vi "GUI AC Source setup.vi"(11 "AC Source":T2) -> (3 "AC Source out":T2)   [LabVIEW 2020]
doc: "Use this template to build a producer/consumer design pattern with events to produce queue items. Use this design pattern instead of the User Interface Event Handler pattern for user interfaces when you want to execute code asynchronously in response to an event without slowing the user interface responsiveness."
uses:
  General AC source/Type definitions/AC Source.ctl
  General AC source/Type definitions/AC Source type.ctl
  <vilib>/Utility/error.llb/DialogType.ctl
  <vilib>/Utility/error.llb/Error Cluster From Error Code.vi
  <vilib>/ErrorRing/Error Ring.xnode
  external libraries/varilib/varilib.lvlib
panel:
  out "not tested label":string="This device is not\nyet fully tested!"
  in  "Ref. clock (Hz)":dbl caption="Reference clock (Hz)\nIf set to zero, ref. clock is not used." format="%#_6p"
  in  "AC source type":T1
  in  "VISA":refnum<visa-resource-name>
  out "gui_elements":refnum<vi>[](array[refnum])
  out "Status":string
  in  "save_and_quit":bool
  in  "test":bool
  in  "cancel":bool
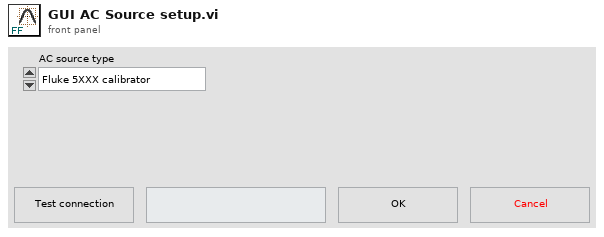
[diagram p1: front panel]
types:
  T1 = typedef "AC Source type.ctl" = enum16{"Fluke 5XXX calibrator", "Tektronix AFG3101C", "dummy"}
  T2 = typedef "AC Source.ctl" = cluster{"AC Source type":T1, "VISA":refnum<visa-resource-name>, "Ref. clock (Hz)":dbl, "status ref":refnum<vi>}
  T3 = typedef "DialogType.ctl" = u16
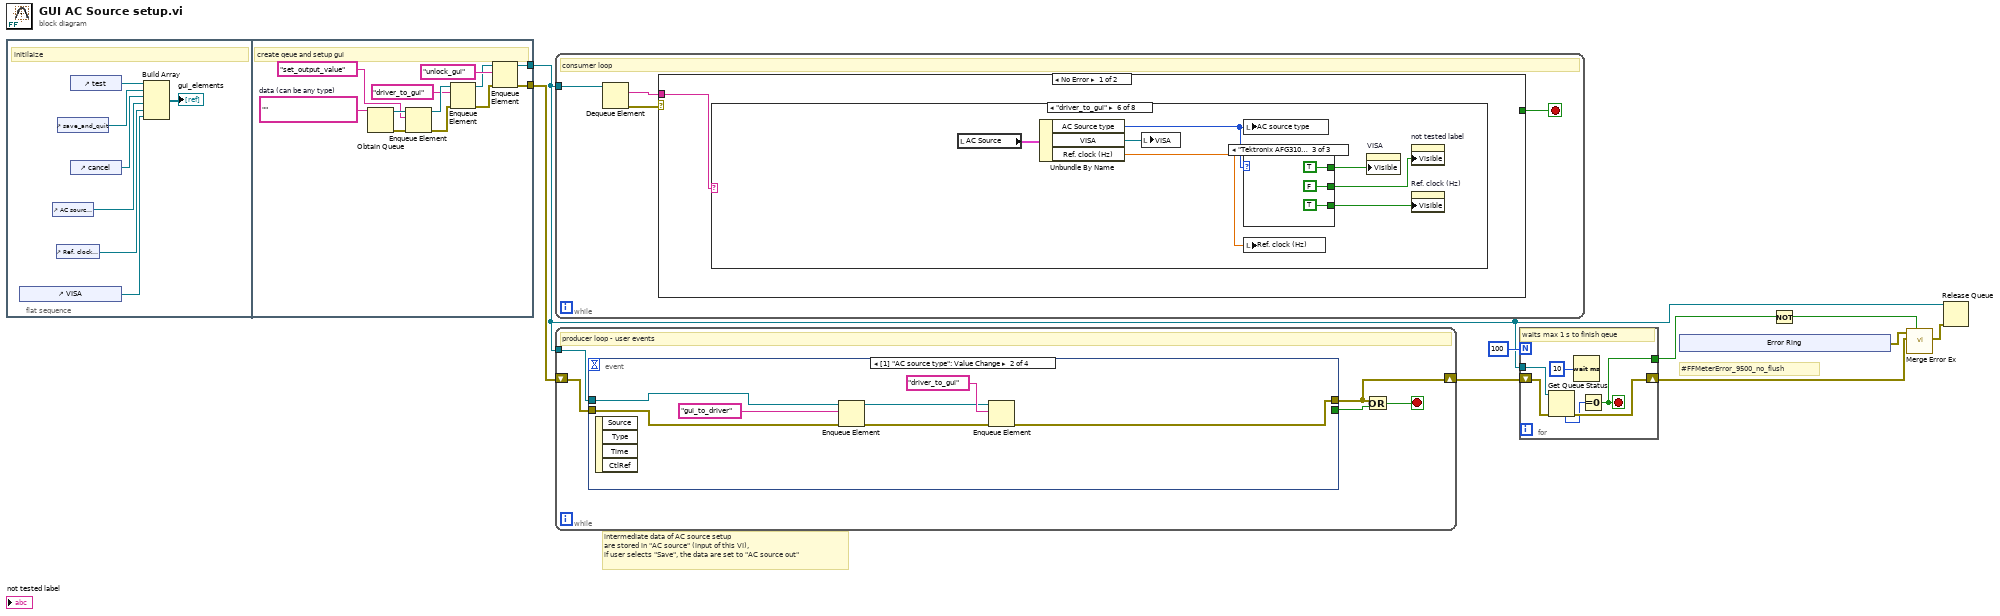
[diagram p0: block diagram]
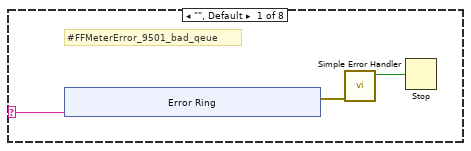
[diagram p2: hidden frame]
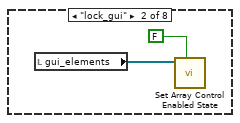
[diagram p3: hidden frame]
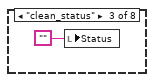
[diagram p4: hidden frame]
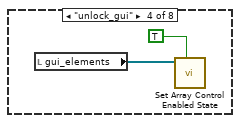
[diagram p5: hidden frame]
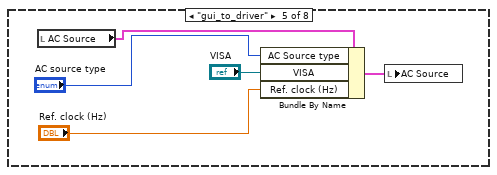
[diagram p6: hidden frame]
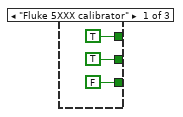
[diagram p7: hidden frame]
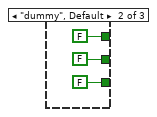
[diagram p8: hidden frame]
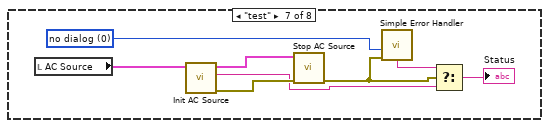
[diagram p9: hidden frame]
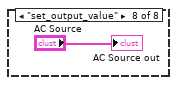
[diagram p10: hidden frame]
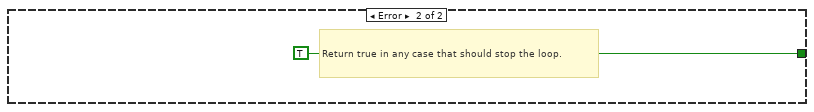
[diagram p11: hidden frame]
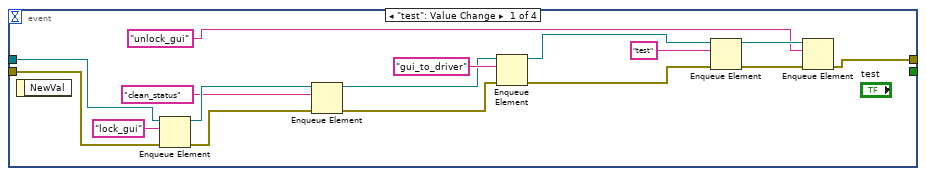
[diagram p12: hidden frame]
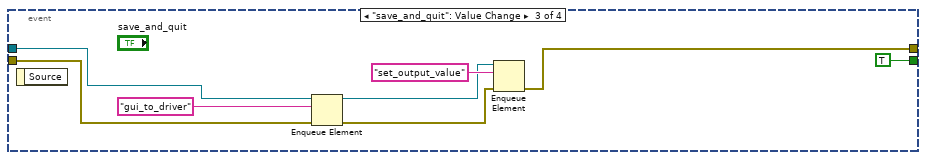
[diagram p13: hidden frame]
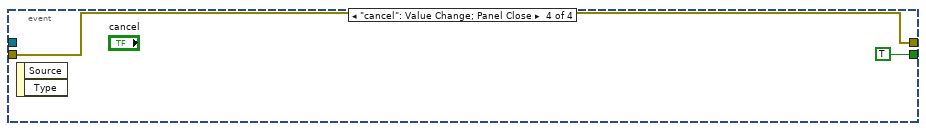
[diagram p14: hidden frame]
diagram:
  # "#FFMeterError_9500_no_flush"
  # "intermediate data of AC source setup\nare stored in \"AC source\" (input of this VI),\nif user selects \"Save\", the data are set to \"AC source out\""
  n1 = flat-sequence {
    tunnel: [w21] -> w2
    tunnel: [w19] -> w1
    frame #0 {
      # "initilaize"
      n2 = control-ref of="VISA"() -> (w12:refnum<vi>)
      n3 = control-ref of="AC source type"() -> (w11:refnum<vi>)
      n4 = control-ref of="Ref. clock (Hz)"() -> (w10:refnum<vi>)
      n5 = control-ref of="save_and_quit"() -> (w15:refnum<vi>)
      n6 = control-ref of="test"() -> (w16:refnum<vi>)
      n7 = control-ref of="cancel"() -> (w14:refnum<vi>)
      n8 = Build Array(w16, w15, w14, w11, w10, w12) -> (→"gui_elements":refnum<vi>[])
    }
    frame #1 {
      w20 = ""  # data (can be any type)
      # "create qeue and setup gui"
      n9 = Obtain Queue(element data type=w20) -> (queue out=w25:refnum<queue>, error out=w27:errorcluster)  [unwired: 4 in, 1 out]
      n10 = Enqueue Element(queue=w25, element="set_output_value", error in (no error)=w27) -> (queue out=w26:refnum<queue>, error out=w28:errorcluster)  [unwired: 1 in, 1 out]
      n11 = Enqueue Element(queue=w26, element="driver_to_gui", error in (no error)=w28) -> (queue out=w17:refnum<queue>, error out=w18:errorcluster)  [unwired: 1 in, 1 out]
      n12 = Enqueue Element(queue=w17, element="unlock_gui", error in (no error)=w18) -> (queue out=w21:refnum<queue>, error out=w19:errorcluster)  [unwired: 1 in, 1 out]
    }
  }
  n13 = while {
    tunnel: w2 -> [w32]
    stop <- w29 stop-if-true
    # "consumer loop"
    n14 = Dequeue Element(queue=w32) -> (element=w30:string, error out=w31:errorcluster)  [unwired: 2 in, 2 out]
    n15 = case shown="No Error" w31 {
      tunnel: w30 -> [w33 _]
      tunnel: [_ TRUE] -> w29
      frame No Error {
        n16 = case shown="\"driver_to_gui\"" w33 {
          selector: w33 -> [w34 _ _ _ _ _ _ _]
          frame "", Default {
            # "#FFMeterError_9501_bad_qeue"
            n17 = xnode "Error Ring"("parameter 0"=w34) -> ("error out"=w36:errorcluster)
            n18 = call <vilib>:"Simple Error Handler.vi"("error in (no error)"=w36) -> ("error?"=w35:bool)  [unwired: 4 in, 4 out]
            n19 = Stop(stop? (T)=w35) -> ()
          }
          frame "lock_gui" {
            n20 = local read "gui_elements"() -> (w45:refnum<vi>[])
            n21 = call "Set Array Control Enabled State.vi"("enabled (T)"=FALSE, "reference array in"=w45) -> ()  [unwired: 8 in, 2 out]
          }
          frame "clean_status" {
            n22 = local write "Status"("") -> ()
          }
          frame "unlock_gui" {
            n23 = local read "gui_elements"() -> (w48:refnum<vi>[])
            n24 = call "Set Array Control Enabled State.vi"("enabled (T)"=TRUE, "reference array in"=w48) -> ()  [unwired: 8 in, 2 out]
          }
          frame "gui_to_driver" {
            n25 = local read "AC Source"() -> (w52:T2)
            n26 = Bundle By Name(cluster=w52, "AC Source type"="AC source type", "VISA"="VISA", "Ref. clock (Hz)"="Ref. clock (Hz)") -> (w53:T2)
            n27 = local write "AC Source"(w53) -> ()
          }
          frame "driver_to_gui" {
            n28 = local read "AC Source"() -> (w60:T2)
            n29 = Unbundle By Name(w60) -> ("AC Source type"=w59:T1, "VISA"=w56:refnum<visa-resource-name>, "Ref. clock (Hz)"=w58:dbl)
            n30 = local write "VISA"(w56) -> ()
            n31 = local write "AC source type"(w59) -> ()
            n32 = case shown="\"Tektronix AFG3101C\"" w59 {
              tunnel: [FALSE ("x") FALSE ("x") TRUE ("x")] -> w55
              tunnel: [TRUE ("x") FALSE ("x") TRUE ("x")] -> w57
              tunnel: [TRUE ("x") FALSE ("x") FALSE ("x")] -> w54
              frame "Fluke 5XXX calibrator" {
              }
              frame "dummy", Default {
              }
              frame "Tektronix AFG3101C" {
              }
            }
            n33 = local write "Ref. clock (Hz)"(w58) -> ()
            n34 = property on="VISA" class="VISAName"("Visible"=w57) -> ()  [unwired: 2 in, 2 out]
            n35 = property on="not tested label" class="Str"("Visible"=w54) -> ()  [unwired: 2 in, 2 out]
            n36 = property on="Ref. clock (Hz)" class="DigNum (strict)"("Visible"=w55) -> ()  [unwired: 2 in, 2 out]
          }
          frame "test" {
            w77 = T3 0 items=["no dialog", "OK message", "continue or stop message", "OK message + warnings", "continue/stop + warnings"] ("type of dialog (OK msg:1)")
            n37 = local read "AC Source"() -> (w74:T2)
            n38 = call "Init AC Source.vi"("AC source"=w74) -> ("error out"=w72:errorcluster, "Init status"=w71:string, "AC source out"=w73:T2)  [unwired: 8 in]
            n39 = call "Stop AC Source.vi"("error in (no error)"=w72, "AC source"=w73) -> ("error out"=w70:errorcluster)  [unwired: 8 in, 1 out]
            n40 = call <vilib>:"Simple Error Handler.vi"("type of dialog (OK msg:1)"=w77, "error in (no error)"=w70) -> ("message"=w76:string)  [unwired: 3 in, 4 out]
            n41 = Select(t=w76, s=w70, f=w71) -> (s? t:f=→"Status":string)
          }
          frame "set_output_value" {
            "AC Source out" <- "AC Source"
          }
        }
      }
      frame Error {
        # "Return true in any case that should stop the loop."
      }
    }
  }
  n42 = while {
    shift-right: [w80] -> w5
    shift-left: w1 -> [w83]
    tunnel: w2 -> [w84]
    stop <- w81 stop-if-true
    # "producer loop - user events"
    n43 = event shown="[1] \"AC source type\": Value Change" {
      selector: _ -> [_ _ _ _]
      dyn-events: _ -> [_ _ _ _]
      timeout: _ -> [_ _ _ _]
      tunnel: w84 -> [w91 w106 w112 _]
      tunnel: w83 -> [w92 w103 w109 w117]
      tunnel: [w95 w101 w108 w117] -> w80
      tunnel: [_ _ TRUE ("cancel") TRUE ("cancel")] -> w82
      event "test": Value Change {
        n44 = event-data() -> ()  [unwired: 1 in, 1 out]
        n45 = Enqueue Element(queue=w91, element="lock_gui", error in (no error)=w92) -> (queue out=w88:refnum<queue>, error out=w89:errorcluster)  [unwired: 1 in, 1 out]
        n46 = Enqueue Element(queue=w88, element="clean_status", error in (no error)=w89) -> (queue out=w86:refnum<queue>, error out=w87:errorcluster)  [unwired: 1 in, 1 out]
        n47 = Enqueue Element(queue=w86, element="gui_to_driver", error in (no error)=w87) -> (queue out=w98:refnum<queue>, error out=w99:errorcluster)  [unwired: 1 in, 1 out]
        n48 = Enqueue Element(queue=w98, element="test", error in (no error)=w99) -> (queue out=w94:refnum<queue>, error out=w96:errorcluster)  [unwired: 1 in, 1 out]
        n49 = Enqueue Element(queue=w94, element="unlock_gui", error in (no error)=w96) -> (error out=w95:errorcluster)  [unwired: 1 in, 2 out]
      }
      event Value Change {
        n50 = event-data() -> ()  [unwired: 1 in, 4 out]
        n51 = Enqueue Element(queue=w106, element="gui_to_driver", error in (no error)=w103) -> (queue out=w104:refnum<queue>, error out=w102:errorcluster)  [unwired: 1 in, 1 out]
        n52 = Enqueue Element(queue=w104, element="driver_to_gui", error in (no error)=w102) -> (error out=w101:errorcluster)  [unwired: 1 in, 2 out]
      }
      event "save_and_quit": Value Change {
        n53 = event-data() -> ()  [unwired: 1 in, 1 out]
        n54 = Enqueue Element(queue=w112, element="gui_to_driver", error in (no error)=w109) -> (queue out=w111:refnum<queue>, error out=w110:errorcluster)  [unwired: 1 in, 1 out]
        n55 = Enqueue Element(queue=w111, element="set_output_value", error in (no error)=w110) -> (error out=w108:errorcluster)  [unwired: 1 in, 2 out]
      }
      event "cancel": Value Change; Panel Close {
        n56 = event-data() -> ()  [unwired: 1 in, 2 out]
      }
    }
    n57 = Or(x=w80, y=w82) -> (x .or. y?=w81:bool)
  }
  n58 = for {
    N: 100 -> [_]
    tunnel: w2 -> [w123]
    shift-right: [w121] -> w6
    shift-left: w5 -> [w122]
    tunnel: [w118] -> w3
    stop <- w118 stop-if-true
    # "waits max 1 s to finish qeue"
    n59 = Get Queue Status(queue=w123, error in (no error)=w122) -> (error out=w121:errorcluster, # elements in queue=w119:i32)  [unwired: 1 in, 6 out]
    n60 = Wait (ms)(milliseconds to wait=u32 10) -> ()  [unwired: 1 out]
    n61 = Equal To 0?(x=w119) -> (x = 0?=w118:bool)
  }
  n62 = xnode "Error Ring"() -> ("error out"=w7:errorcluster)
  n63 = Not(x=w3) -> (.not. x?=w8:bool)
  n64 = call "Merge Error Ex.vi"("Is error? (False)"=w8, "main error in (no error)"=w6, "second error in"=w7) -> ("error out"=w4:errorcluster)  [unwired: 8 in]
  n65 = Release Queue(queue=w2, error in (no error)=w4) -> ()  [unwired: 1 in, 3 out]
